vi "RyanChargeDischargeCycling.vi"() -> ()   [LabVIEW 2020]
uses:
  <instrlib>/NH Research Regenerative Test Series/Public/Configure/Output Safety.ctl
  <vilib>/DAQmx/read.llb/DAQmx Read (Analog 1D DBL NChan 1Samp).vi
  <vilib>/DAQmx/miscellaneous.llb/DAQmx Fill In Error Info.vi
  <instrlib>/NH Research Regenerative Test Series/Public/Data/Read (Ave Current).vi
  <instrlib>/NH Research Regenerative Test Series/Public/Data/Low Level/Fetch (Ave Voltage).vi
  <instrlib>/NH Research Regenerative Test Series/Public/Data/Low Level/Fetch (Ave True Power).vi
  <instrlib>/NH Research Regenerative Test Series/NH Research Regenerative Test Series.lvlib
panel:
  in  "Discharge Current":dbl
  out "Loop Count":dbl
  in  "Loop Number":dbl
  in  "Discharge Voltage Setpoint":dbl
  out "Task error out":errorcluster
  out "String":string
  out "Filename Out 3":path caption="Filename Out"
  in  "Path 3":path
  out "Ave Current (A) 3":dbl
  out "Ave Voltage (V) 3":dbl
  out "Ave True Power (W) 3":dbl
  out "Status Byte Register 3":T1
  out "Voltage Compare":dbl
  out "BatteryWaterIn 2":dbl
  out "BatteryWaterOut 2":dbl
  out "BatteryTempExt 2":dbl
  out "BatteryTempInternal 2":dbl
  in  "Wait time":dbl
  out "Filename Out 2":path caption="Filename Out"
  in  "Path 2":path
  out "Ave Current (A) 2":dbl
  out "Ave Voltage (V) 2":dbl
  out "Ave True Power (W) 2":dbl
  out "Status Byte Register 2":T1
  out "WaitElapsed Time (s)":dbl caption="Elapsed Time (s)"
  in  "Output Safety":T2
  out "Filename Out":path
  in  "DAQmx Task Name":refnum<k21>
  in  "Path":path
  in  "Charge Current Cutoff":dbl
  out "Ave Current (A)":dbl
  out "Ave Voltage (V)":dbl
  out "Ave True Power (W)":dbl
  out "Status Byte Register":T1
  out "Current Compare":dbl
  out "BatteryWaterIn":dbl
  out "BatteryWaterOut":dbl
  out "BatteryTempExt":dbl
  out "BatteryTempInternal":dbl
  in  "Logical Instrument Number":u32=1
  in  "Charge Current":dbl format="%#.6g"
  in  "Charge Voltage":dbl format="%#.6g"
  in  "Battery Detect Voltage (0V)":dbl format="%#.6g"
  in  "VISA resource name":refnum<visa-resource-name>
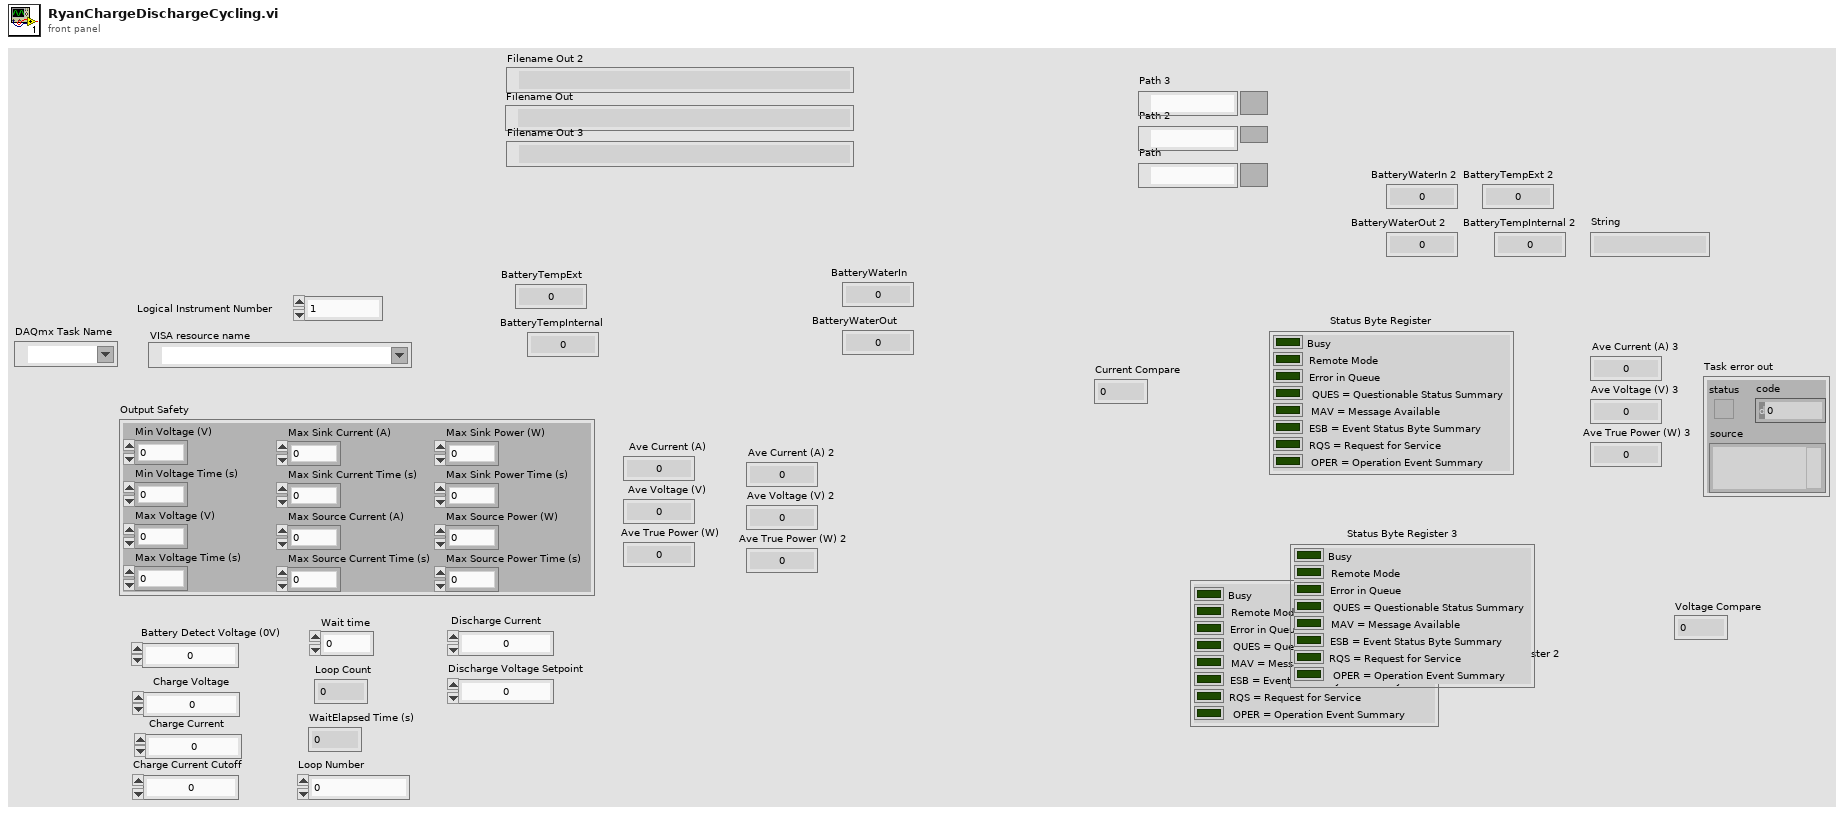
[diagram p1: front panel]
types:
  T1 = cluster{"Busy":bool, "Remote Mode":bool, "Error in Queue":bool, "QUES = Questionable Status Summary":bool, "MAV = Message Available":bool, "ESB = Event Status Byte Summary":bool, "RQS = Request for Service":bool, "OPER = Operation Event Summary":bool}
  T2 = typedef "NH Research Regenerative Test Series.lvlib/Output Safety.ctl" = cluster{"Min Voltage (V)":dbl, "Min Voltage Time (s)":dbl, "Max Voltage (V)":dbl, "Max Voltage Time (s)":dbl, "Max Sink Current (A)":dbl, "Max Sink Current Time (s)":dbl, "Max Source Current (A)":dbl, "Max Source Current Time (s)":dbl, "Max Sink Power (W)":dbl, "Max Sink Power Time (s)":dbl, "Max Source Power (W)":dbl, "Max Source Power Time (s)":dbl}
  T3 = cluster{"data[0]":dbl, "data[1]":dbl, "data[2]":dbl, "data[3]":dbl, "data[4]":dbl, "data[5]":dbl, "data[6]":dbl, "data[7]":dbl, "data[8]":dbl}
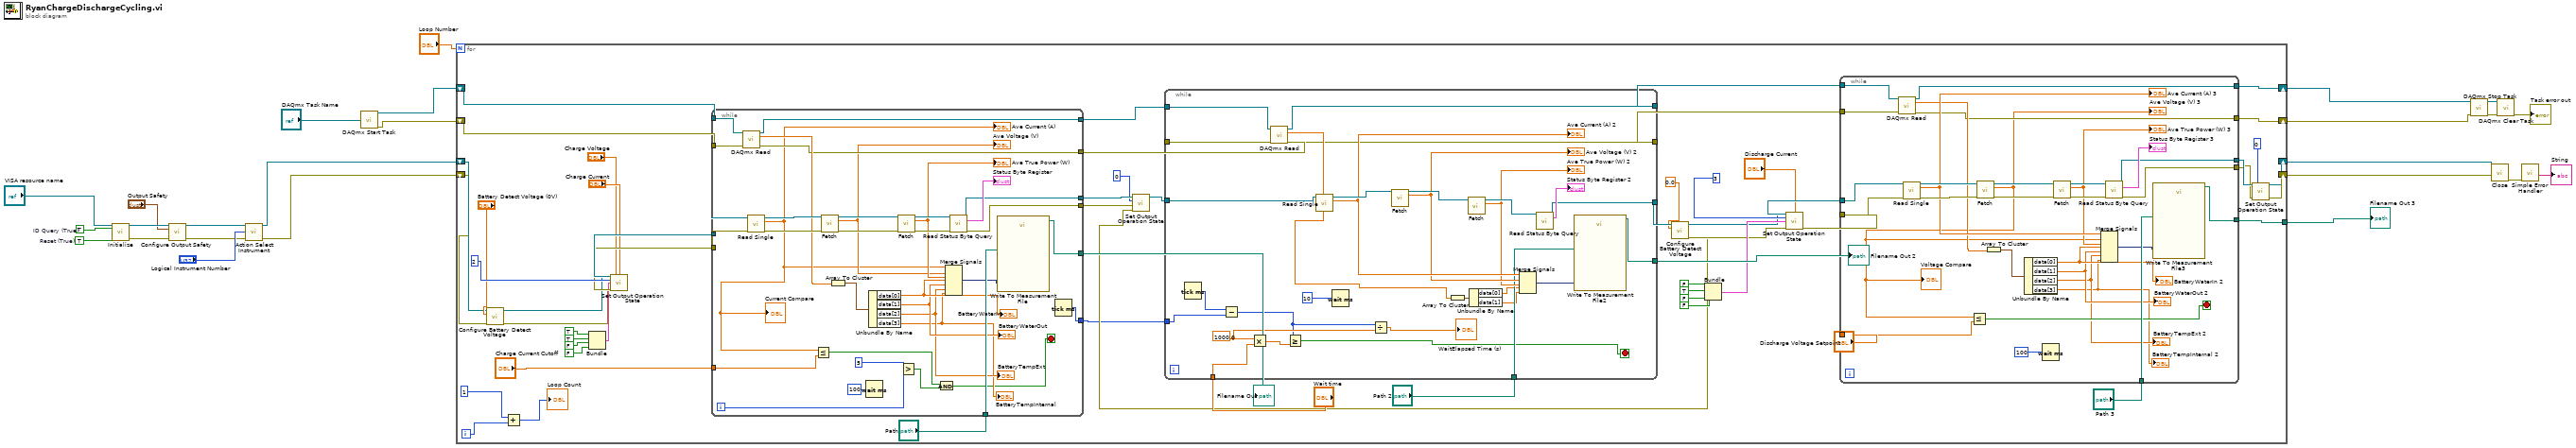
[diagram p0: block diagram]
diagram:
  w24 = TRUE  # ID Query (True)
  w23 = TRUE  # Reset (True)
  n1 = call <vilib>:"Initialize.vi"("VISA resource name"="VISA resource name", "ID Query (True)"=w24, "Reset (True)"=w23) -> ("VISA resource name out"=w22:refnum<visa-resource-name>, "error out"=w21:errorcluster)  [unwired: 11 in]
  n2 = call <vilib>:"Configure Output Safety.vi"("VISA resource name"=w22, "Output Safety"="Output Safety", "error in (no error)"=w21) -> ("VISA resource name out"=w18:refnum<visa-resource-name>, "error out"=w14:errorcluster)  [unwired: 11 in]
  n3 = call <instrlib>:"Action Select Instrument.vi"("VISA resource name"=w18, "Logical Instrument Number"="Logical Instrument Number", "error in (no error)"=w14) -> ("VISA resource name out"=w2:refnum<visa-resource-name>, "error out"=w1:errorcluster)  [unwired: 11 in]
  n4 = call <vilib>:"DAQmx Start Task.vi"("task/channels in"="DAQmx Task Name") -> ("task out"=w16:refnum<k21>, "error out"=w15:errorcluster)  [unwired: 13 in]
  n5 = for {
    N: "Loop Number" -> [_]
    tunnel: [w73] -> w13
    shift-right: [w55] -> w3
    shift-left: w2 -> [w33]
    shift-right: [w56] -> w4
    shift-left: w1 -> [w31]
    shift-right: [w72] -> w7
    shift-left: w16 -> [w82]
    shift-right: [w71] -> w6
    shift-left: w15 -> [w81]
    i -> [w27]
    n6 = call <vilib>:"Configure Battery Detect Voltage.vi"("VISA resource name"=w33, "Battery Detect Voltage (0V)"="Battery Detect Voltage (0V)", "error in (no error)"=w31) -> ("VISA resource name out"=w32:refnum<visa-resource-name>, "error out"=w30:errorcluster)  [unwired: 11 in]
    n7 = Add(x=1, y=w27) -> (x+y=→"Loop Count":i32)
    n8 = Bundle(TRUE, TRUE, FALSE, FALSE) -> (w34:cluster{bool, bool, bool, bool})  [unwired: 1 in]
    n9 = call <vilib>:"Set Output Operation State.vi"("VISA resource name"=w32, "Voltage Setpoint (0 V)"="Charge Voltage", "Current Setpoint (0 A)"="Charge Current", "Mode (0: Off)"=2, "Enable"=w34, "error in (no error)"=w30) -> ("VISA resource name out"=w43:refnum<visa-resource-name>, "error out"=w42:errorcluster)  [unwired: 8 in]
    n10 = while {
      tunnel: w43 -> [w172]
      tunnel: w42 -> [w171]
      tunnel: [w169] -> w50
      tunnel: [w168] -> w49
      tunnel: "Charge Current Cutoff" -> [w157]
      tunnel: "Path" -> [w166]
      tunnel: w82 -> [w165]
      tunnel: [w161] -> w76
      tunnel: [w160] -> w75
      tunnel: w81 -> [w159]
      tunnel: [w158] -> w83
      tunnel: [w144] -> w29
      i -> [w145]
      stop <- w148 stop-if-true
      n11 = call-poly <vilib>:"DAQmx Read.vi"("task/channels in"=w165, "error in"=w159) -> ("task out"=w161:refnum<k21>, "data"=w164:dbl[], "error out"=w160:errorcluster)  [unwired: 11 in]
      n12 = call-poly <instrlib>:"Read Single.vi"("VISA resource name"=w172, "error in (no error)"=w171) -> ("VISA resource name out"=w177:refnum<visa-resource-name>, "Ave Current (A)"=w151:dbl, "error out"=w178:errorcluster)  [unwired: 11 in]
      "Ave Current (A)" <- w151
      "Current Compare" <- w151
      n13 = Less Or Equal?(x=w151, y=w157) -> (x <= y?=w147:bool)
      n14 = call-poly <instrlib>:"Fetch.vi"("VISA resource name"=w177, "error in (no error)"=w178) -> ("VISA resource name out"=w176:refnum<visa-resource-name>, "Ave Voltage (V)"=w156:dbl, "error out"=w175:errorcluster)  [unwired: 11 in]
      "Ave Voltage (V)" <- w156
      n15 = Array To Cluster(array=w164) -> (cluster=w163:T3)
      n16 = Wait (ms)(milliseconds to wait=100) -> ()  [unwired: 1 out]
      n17 = Unbundle By Name(w163) -> ("data[0]"=w155:dbl, "data[1]"=w154:dbl, "data[2]"=w153:dbl, "data[3]"=w152:dbl)
      "BatteryWaterIn" <- w155
      "BatteryWaterOut" <- w154
      "BatteryTempExt" <- w153
      "BatteryTempInternal" <- w152
      n18 = call-poly <instrlib>:"Fetch.vi"("VISA resource name"=w176, "error in (no error)"=w175) -> ("VISA resource name out"=w174:refnum<visa-resource-name>, "Ave True Power (W)"=w167:dbl, "error out"=w173:errorcluster)  [unwired: 11 in]
      "Ave True Power (W)" <- w167
      n19 = Greater?(x=w145, y=5) -> (0:w146:bool)
      n20 = And(x=w147, y=w146) -> (x .and. y?=w148:bool)
      n21 = Merge Signals "Merge Signals"(w151, w156, w167, w155, w154, w153, w152) -> (w162:dynamicdata)
      n22 = call <instrlib>:"Read Status Byte Query.vi"("VISA resource name"=w174, "error in (no error)"=w173) -> ("VISA resource name out"=w169:refnum<visa-resource-name>, "Status Byte Register"=→"Status Byte Register":T1, "error out"=w168:errorcluster)  [unwired: 11 in]
      n23 = call "Write To Measurement File"("Signals"=w162, "Filename"=w166) -> ("Filename Out"=w158:path)  [unwired: 15 in, 2 out]
      n24 = Tick Count (ms)() -> (millisecond timer value=w144:u32)
    }
    "Filename Out" <- w83
    n25 = call <vilib>:"Set Output Operation State.vi"("VISA resource name"=w50, "Mode (0: Off)"=0, "error in (no error)"=w49) -> ("VISA resource name out"=w46:refnum<visa-resource-name>, "error out"=w48:errorcluster)  [unwired: 11 in]
    n26 = while {
      tunnel: [w138] -> w53
      tunnel: "Wait time" -> [w128]
      tunnel: "Path 2" -> [w134]
      tunnel: w29 -> [w118]
      tunnel: [w126] -> w67
      tunnel: [w125] -> w68
      tunnel: w75 -> [w119]
      tunnel: [w124] -> w78
      tunnel: w76 -> [w123]
      tunnel: w46 -> [w122]
      stop <- w129 stop-if-true
      w120 = 1000.0
      n27 = Tick Count (ms)() -> (millisecond timer value=w117:u32)
      n28 = Subtract(x=w117, y=w118) -> (x-y=w116:u32)
      n29 = Multiply(x=w120, y=w128) -> (x*y=w127:dbl)
      n30 = call-poly <vilib>:"DAQmx Read.vi"("task/channels in"=w123, "error in"=w119) -> ("task out"=w125:refnum<k21>, "data"=w133:dbl[], "error out"=w126:errorcluster)  [unwired: 11 in]
      n31 = Greater Or Equal?(x=w116, y=w127) -> (x >= y?=w129:bool)
      n32 = call-poly <instrlib>:"Read Single.vi"("VISA resource name"=w122) -> ("VISA resource name out"=w142:refnum<visa-resource-name>, "Ave Current (A)"=w137:dbl)  [unwired: 12 in, 1 out]
      "Ave Current (A) 2" <- w137
      n33 = Wait (ms)(milliseconds to wait=10) -> ()  [unwired: 1 out]
      n34 = Divide(x=w116, y=w120) -> (x/y=→"WaitElapsed Time (s)":dbl)
      n35 = call-poly <instrlib>:"Fetch.vi"("VISA resource name"=w142) -> ("VISA resource name out"=w141:refnum<visa-resource-name>, "Ave Voltage (V)"=w136:dbl)  [unwired: 12 in, 1 out]
      "Ave Voltage (V) 2" <- w136
      n36 = Array To Cluster(array=w133) -> (cluster=w132:T3)
      n37 = call-poly <instrlib>:"Fetch.vi"("VISA resource name"=w141) -> ("VISA resource name out"=w140:refnum<visa-resource-name>, "Ave True Power (W)"=w135:dbl)  [unwired: 12 in, 1 out]
      "Ave True Power (W) 2" <- w135
      n38 = Unbundle By Name(w132) -> ("data[0]"=w131:dbl, "data[1]"=w130:dbl)
      n39 = Merge Signals "Merge Signals"(w137, w136, w135, w131, w130) -> (w143:dynamicdata)
      n40 = call <instrlib>:"Read Status Byte Query.vi"("VISA resource name"=w140) -> ("VISA resource name out"=w138:refnum<visa-resource-name>, "Status Byte Register"=→"Status Byte Register 2":T1)  [unwired: 12 in, 1 out]
      n41 = call "Write To Measurement File2"("Signals"=w143, "Filename"=w134) -> ("Filename Out"=w124:path)  [unwired: 15 in, 2 out]
    }
    "Filename Out 2" <- w78
    n42 = call <vilib>:"Configure Battery Detect Voltage.vi"("VISA resource name"=w53, "Battery Detect Voltage (0V)"=0.0, "error in (no error)"=w48) -> ("VISA resource name out"=w52:refnum<visa-resource-name>, "error out"=w54:errorcluster)  [unwired: 11 in]
    n43 = Bundle(FALSE, TRUE, FALSE, FALSE) -> (w61:cluster{bool, bool, bool, bool})  [unwired: 1 in]
    n44 = call <vilib>:"Set Output Operation State.vi"("VISA resource name"=w52, "Current Setpoint (0 A)"="Discharge Current", "Mode (0: Off)"=3, "Enable"=w61, "error in (no error)"=w54) -> ("VISA resource name out"=w69:refnum<visa-resource-name>, "error out"=w70:errorcluster)  [unwired: 9 in]
    n45 = while {
      tunnel: w69 -> [w108]
      tunnel: w70 -> [w107]
      tunnel: [w105] -> w59
      tunnel: [w104] -> w58
      tunnel: "Discharge Voltage Setpoint" -> [w91]
      tunnel: "Path 3" -> [w101]
      tunnel: w68 -> [w100]
      tunnel: [w96] -> w72
      tunnel: [w95] -> w71
      tunnel: w67 -> [w94]
      tunnel: [w93] -> w73
      stop <- w92 stop-if-true
      n46 = call-poly <vilib>:"DAQmx Read.vi"("task/channels in"=w100, "error in"=w94) -> ("task out"=w96:refnum<k21>, "data"=w99:dbl[], "error out"=w95:errorcluster)  [unwired: 11 in]
      n47 = call-poly <instrlib>:"Read Single.vi"("VISA resource name"=w108, "error in (no error)"=w107) -> ("VISA resource name out"=w113:refnum<visa-resource-name>, "Ave Current (A)"=w103:dbl, "error out"=w114:errorcluster)  [unwired: 11 in]
      "Ave Current (A) 3" <- w103
      n48 = call-poly <instrlib>:"Fetch.vi"("VISA resource name"=w113, "error in (no error)"=w114) -> ("VISA resource name out"=w112:refnum<visa-resource-name>, "Ave Voltage (V)"=w90:dbl, "error out"=w111:errorcluster)  [unwired: 11 in]
      "Ave Voltage (V) 3" <- w90
      "Voltage Compare" <- w90
      n49 = Less Or Equal?(x=w90, y=w91) -> (x <= y?=w92:bool)
      n50 = Array To Cluster(array=w99) -> (cluster=w98:T3)
      n51 = Unbundle By Name(w98) -> ("data[0]"=w89:dbl, "data[1]"=w88:dbl, "data[2]"=w87:dbl, "data[3]"=w86:dbl)
      "BatteryWaterIn 2" <- w89
      "BatteryWaterOut 2" <- w88
      "BatteryTempExt 2" <- w87
      "BatteryTempInternal 2" <- w86
      n52 = Wait (ms)(milliseconds to wait=100) -> ()  [unwired: 1 out]
      n53 = call-poly <instrlib>:"Fetch.vi"("VISA resource name"=w112, "error in (no error)"=w111) -> ("VISA resource name out"=w110:refnum<visa-resource-name>, "Ave True Power (W)"=w102:dbl, "error out"=w109:errorcluster)  [unwired: 11 in]
      "Ave True Power (W) 3" <- w102
      n54 = Merge Signals "Merge Signals"(w103, w90, w102, w89, w88, w87, w86) -> (w97:dynamicdata)
      n55 = call <instrlib>:"Read Status Byte Query.vi"("VISA resource name"=w110, "error in (no error)"=w109) -> ("VISA resource name out"=w105:refnum<visa-resource-name>, "Status Byte Register"=→"Status Byte Register 3":T1, "error out"=w104:errorcluster)  [unwired: 11 in]
      n56 = call "Write To Measurement File3"("Signals"=w97, "Filename"=w101) -> ("Filename Out"=w93:path)  [unwired: 15 in, 2 out]
    }
    n57 = call <vilib>:"Set Output Operation State.vi"("VISA resource name"=w59, "Mode (0: Off)"=0, "error in (no error)"=w58) -> ("VISA resource name out"=w55:refnum<visa-resource-name>, "error out"=w56:errorcluster)  [unwired: 11 in]
  }
  "Filename Out 3" <- w13
  n58 = call <vilib>:"DAQmx Stop Task.vi"("task/channels in"=w7, "error in"=w6) -> ("task out"=w11:refnum<k21>, "error out"=w10:errorcluster)  [unwired: 12 in]
  n59 = call <instrlib>:"Close.vi"("VISA resource name"=w3, "error in (no error)"=w4) -> ("error out"=w8:errorcluster)  [unwired: 13 in]
  n60 = call <vilib>:"DAQmx Clear Task.vi"("task in"=w11, "error in"=w10) -> ("error out"=→"Task error out":errorcluster)  [unwired: 13 in]
  n61 = call <vilib>:"Simple Error Handler.vi"("error in (no error)"=w8) -> ("source out"=→"String":string)  [unwired: 4 in, 4 out]
